vi "SubVI1.vi"(9 "x":dbl) -> (0 "x+y":dbl)   [LabVIEW 2022 SP3]
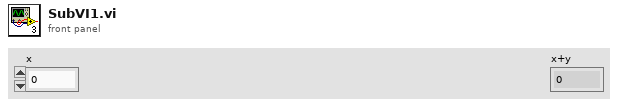
[diagram p1: front panel]
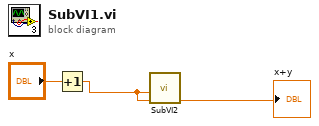
[diagram p0: block diagram]
diagram:
  n1 = Increment(x="x") -> (x+1=w2:dbl)
  n2 = call "SubVI2.vi"("y"=w2, "x"=w2) -> ("x+y"=→"x+y":dbl)  [unwired: 9 in]
